vi "UTC_time_stamp_V2.vi"() -> ()   [LabVIEW 2017]
panel:
  out "Timestamp":timestamp
  in  "error in":errorcluster
  out "error out":errorcluster
  out "ISO-8601 UTC Formatted DateTime String":string
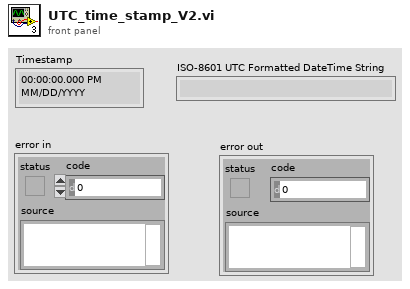
[diagram p1: front panel]
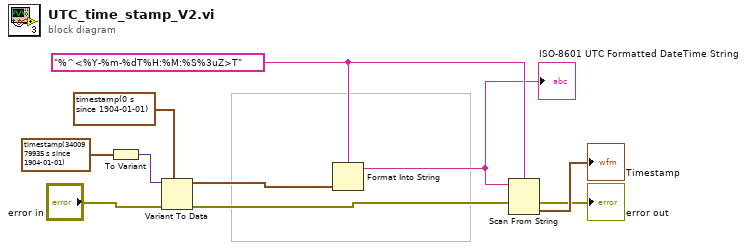
[diagram p0: block diagram]
diagram:
  w3 = "%^<%Y-%m-%dT%H:%M:%S%3uZ>T" ("format string")
  n1 = To Variant(anything=timestamp(3400979935.297035 s since 1904-01-01) ("time stamp")) -> (Variant=w8:variant)
  n2 = Variant To Data(error in="error in", type=timestamp(0 s since 1904-01-01) ("time stamp"), Variant=w8) -> (data=w2:timestamp, error out=w5:errorcluster)
  n3 = Format Into String(format string=w3, w2) -> (resulting string=w1:string)  [unwired: 2 in, 1 out]
  "ISO-8601 UTC Formatted DateTime String" <- w1
  n4 = Scan From String(format string=w3, input string=w1, error in=w5) -> (error out=→"error out":errorcluster, output 1=→"Timestamp":timestamp)  [unwired: 2 in, 2 out]
